vi "Set & Minimize VI by ref.vi"(0 "LV DEV.lvclass":refnum<class "LV DEV.lvclass">, 5 "VI Refnum":refnum<vi>, 11 "Error in":errorcluster) -> (4 "LV DEV.lvclass":refnum<class "LV DEV.lvclass">, 15 "Error Out":errorcluster)   [LabVIEW 2016, in "LV DEV.lvclass"]
doc: "Get reference of given VI."
uses:
  LV DEV.lvclass
  D:/Navin Workspace/MDI/source code/Document/LV Doc/LV Doc.lvclass
  LV Doc.lvclass/LV Doc.ctl
  property/Write VI Reference.vi
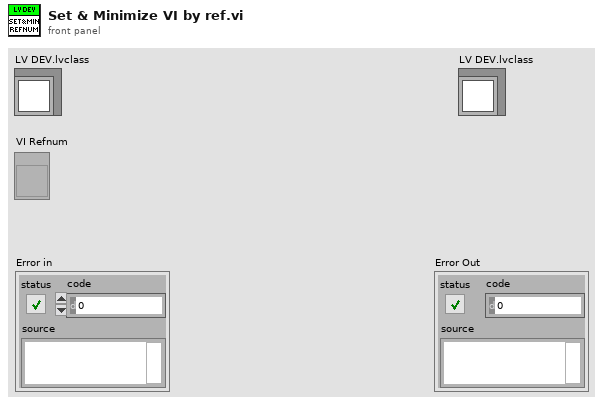
[diagram p1: front panel]
types:
  T1 = enum32{"Invalid", "Standard", "Closed", "Hidden", "Minimized", "Maximized"}
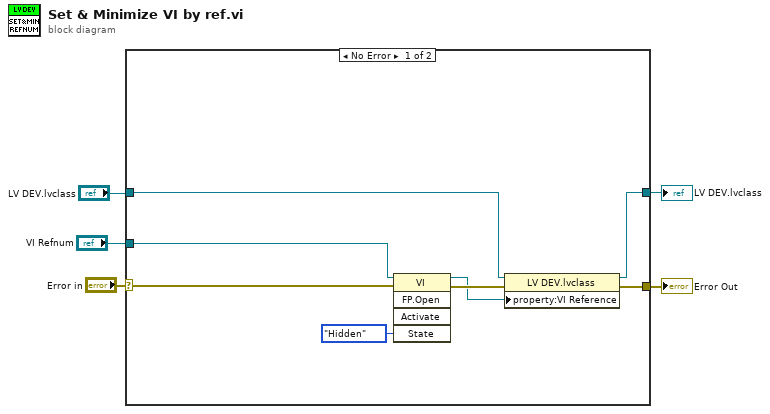
[diagram p0: block diagram]
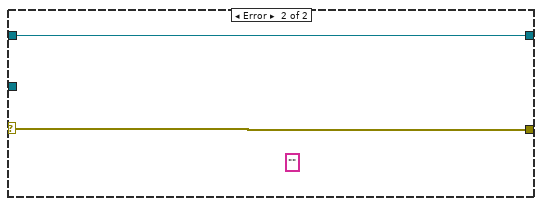
[diagram p2: hidden frame]
diagram:
  n1 = case shown="No Error" "Error in" {
    selector: "Error in" -> [w12 w15]
    tunnel: [w10 w15] -> w4
    tunnel: "LV DEV.lvclass" -> [w11 w14]
    tunnel: [w9 w14] -> w2
    tunnel: "VI Refnum" -> [w6 _]
    frame No Error {
      n2 = invoke class="VI" method="FP.Open"(reference=w6, error in=w12, "State"=T1."Hidden") -> (reference out=w7:refnum<vi>, error out=w8:errorcluster)  [unwired: 2 in, 3 out]
      n3 = property class="LV DEV.lvclass"(reference=w11, error in=w8, "property:VI Reference"=w7) -> (reference out=w9:refnum<class "LV DEV.lvclass">, error out=w10:errorcluster)
    }
    frame Error {
      (unwired) "" ("Front Panel.Title")
    }
  }
  "Error Out" <- w4
  "LV DEV.lvclass" <- w2
